vi "Draw.vi"(8 "error in (no error)":errorcluster, 10 "picture in":picture, 11 "Port in":refnum<class "FSM.Port.lvclass">) -> (0 "error out":errorcluster, 2 "picture out":picture, 3 "Port out":refnum<class "FSM.Port.lvclass">)   [LabVIEW 2015, in "FSM.Port.lvclass"]
uses:
  FSM.Port.lvclass
  FSM.Port.lvclass/FSM.Port.ctl
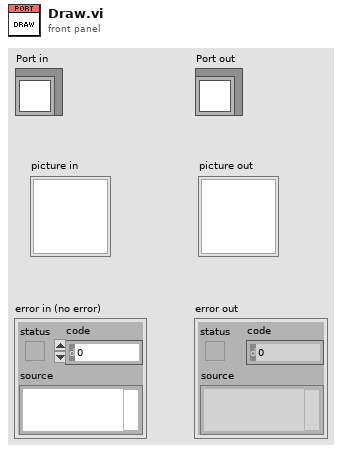
[diagram p1: front panel]
types:
  T1 = cluster{"left":i16, "top":i16, "right":i16, "bottom":i16}
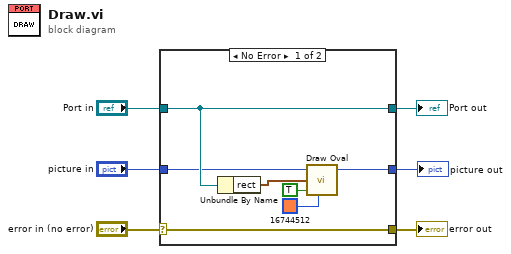
[diagram p0: block diagram]
diagram:
  n1 = case shown="No Error" "error in (no error)" {
    selector: "error in (no error)" -> [w13 w16]
    tunnel: [w13 w16] -> w5
    tunnel: [w12 w15] -> w3
    tunnel: "Port in" -> [w12 w15]
    tunnel: "picture in" -> [w11 w14]
    tunnel: [w10 w14] -> w1
    frame No Error {
      n2 = Unbundle By Name(w12) -> ("rect"=w9:T1)
      n3 = call <vilib>:"Draw Oval.vi"("picture"=w11, "rect"=w9, "fill?(F)"=TRUE, "color(black)"=u32 16744512) -> ("new picture"=w10:picture)  [unwired: 5 in]
    }
    frame Error {
    }
  }
  "error out" <- w5
  "Port out" <- w3
  "picture out" <- w1
